vi "挖开地块.vi"(0 "地图":i32[][](array[numeric]), 1 "索引":i32) -> (2 "输出地图":i32[][](array[numeric]), 3 "对话框信息":string, 4 "胜利失败":bool, 5 "游戏结束":bool)   [LabVIEW 2017]
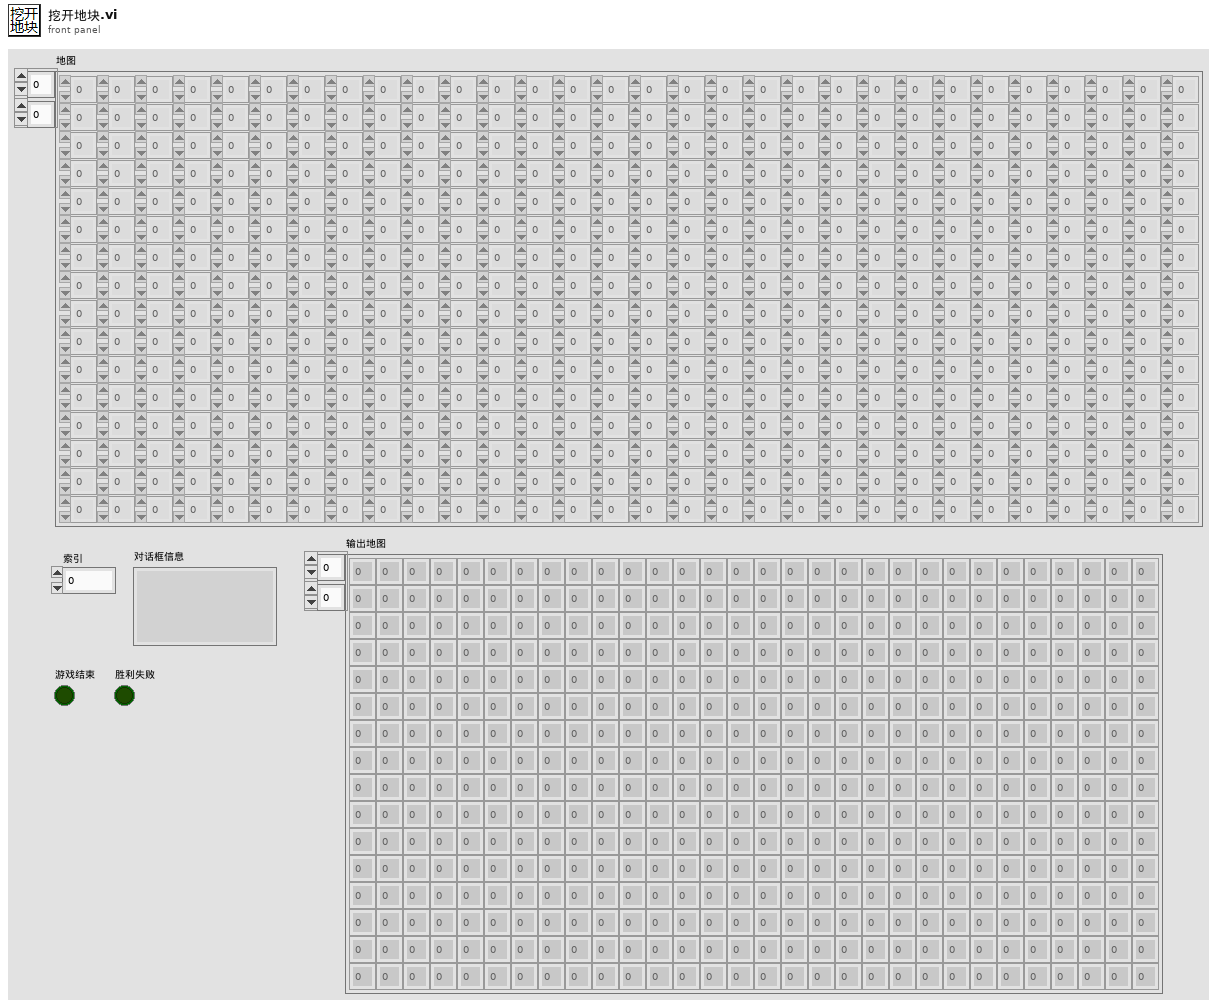
[diagram p1: front panel]
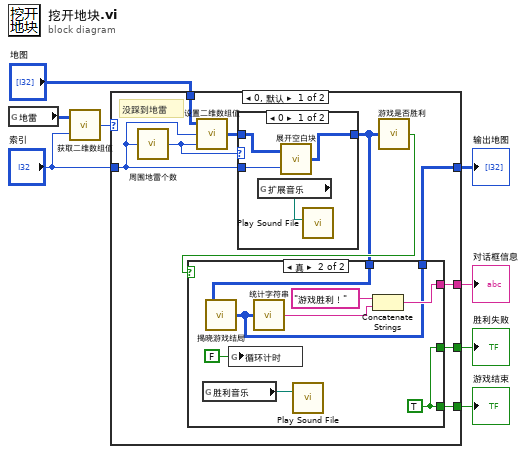
[diagram p0: block diagram]
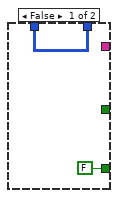
[diagram p3: hidden frame]
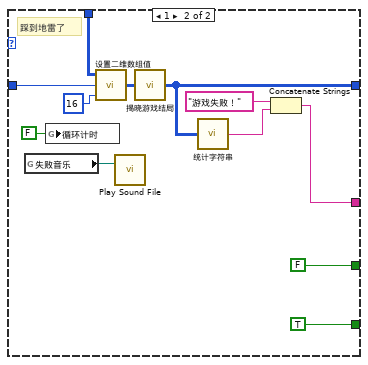
[diagram p4: hidden frame]
diagram:
  n1 = global read "全局变量.vi" "地雷"() -> (w8:i16[][])
  n2 = call "获取二维数组值.vi"("索引"="索引", "数组"=w8) -> ("数值"=w7:i32)
  n3 = case shown="0, 默认" w7 {
    tunnel: "索引" -> [w10 w45]
    tunnel: "地图" -> [w18 w44]
    tunnel: [w16 FALSE] -> w4
    tunnel: [w15 TRUE ("游戏结束")] -> w3
    tunnel: [w14 w41] -> w2
    tunnel: [w13 w38] -> w1
    frame 0, Default {
      # "没踩到地雷"
      n4 = call "周围地雷个数.vi"("索引"=w10) -> ("数值"=w12:i32)
      n5 = call "设置二维数组值.vi"("数值"=w12, "索引"=w10, "数组"=w18) -> ("输出数组"=w11:i32[][])
      n6 = case shown="0" w12 {
        tunnel: w11 -> [w20 w23]
        tunnel: w10 -> [w21 _]
        tunnel: [w19 w23] -> w9
        frame 0 {
          n7 = global read "全局变量.vi" "扩展音乐"() -> (w22:path)
          n8 = call "展开空白块.vi"("索引"=w21, "地图"=w20) -> ("输出地图"=w19:i16[][])
          n9 = call <vilib>:"Play Sound File.vi"("path"=w22) -> ()  [unwired: 9 in, 2 out]
        }
        frame 1, Default {
        }
      }
      n10 = call "游戏是否胜利.vi"("地图"=w9) -> ("胜利"=w17:bool)
      n11 = case shown="真" w17 {
        tunnel: [_ w28] -> w16
        tunnel: [FALSE ("游戏结束") w28] -> w15
        tunnel: [w25 w30] -> w14
        tunnel: [_ w31] -> w13
        tunnel: w9 -> [w25 w29]
        frame False {
        }
        frame True {
          w28 = TRUE ("游戏结束")
          n12 = global read "全局变量.vi" "胜利音乐"() -> (w26:path)
          n13 = call "揭晓游戏结局.vi"("地图"=w29) -> ("输出地图"=w30:i32[][])
          n14 = global write "全局变量.vi" "循环计时"(FALSE ("循环计时")) -> ()
          n15 = call "统计字符串.vi"("地图"=w30) -> ("字符串"=w32:string)
          n16 = call <vilib>:"Play Sound File.vi"("path"=w26) -> ()  [unwired: 9 in, 2 out]
          n17 = Concatenate Strings("游戏胜利！" ("消息"), w32) -> (w31:string)
        }
      }
    }
    frame 1 {
      # "踩到地雷了"
      n18 = global read "全局变量.vi" "失败音乐"() -> (w34:path)
      n19 = global write "全局变量.vi" "循环计时"(FALSE ("循环计时")) -> ()
      n20 = call "设置二维数组值.vi"("数值"=16, "索引"=w45, "数组"=w44) -> ("输出数组"=w42:i32[][])
      n21 = call <vilib>:"Play Sound File.vi"("path"=w34) -> ()  [unwired: 9 in, 2 out]
      n22 = call "揭晓游戏结局.vi"("地图"=w42) -> ("输出地图"=w41:i32[][])
      n23 = call "统计字符串.vi"("地图"=w41) -> ("字符串"=w39:string)
      n24 = Concatenate Strings("游戏失败！" ("消息"), w39) -> (w38:string)
    }
  }
  "游戏结束" <- w3
  "胜利失败" <- w4
  "输出地图" <- w2
  "对话框信息" <- w1
